vi "OAT State Machine Generate Event for Numeric.vi"(1 "Initialize":bool, 2 "Numeric":dbl format="%.2f", 4 "Enum":T1(ring) caption="Action") -> (7 "Event":bool)   [LabVIEW 2017]
doc: "Detects events for the numeric objects. The event of numeric range from changed, zero crossing,sign reversed and so on. When the event detected, the coresponding output is TRUE."
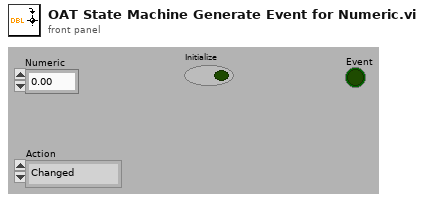
[diagram p1: front panel]
types:
  T1 = enum16{"Changed", ">0 to <0", "<0 to >0", ">0 to <=0", "<=0 to >0", ">=0 to <0", "<0 to >=0", ">0 to =0", "=0 to >0", "<0 to =0", "=0 to <0", "=0", "Zero Crossing", "Sign Reversed"}
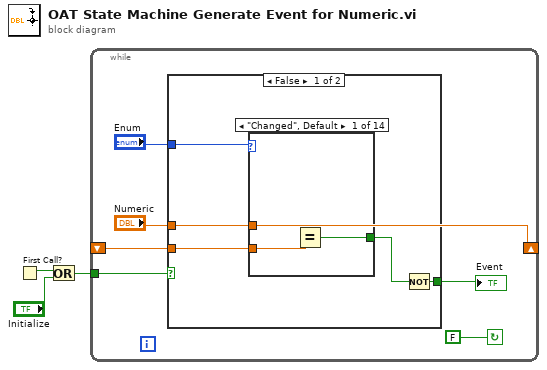
[diagram p0: block diagram]
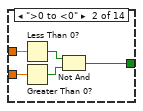
[diagram p2: hidden frame]
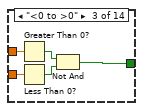
[diagram p3: hidden frame]
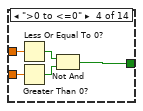
[diagram p4: hidden frame]
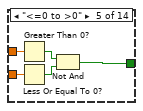
[diagram p5: hidden frame]
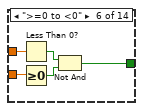
[diagram p6: hidden frame]
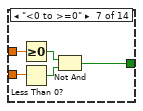
[diagram p7: hidden frame]
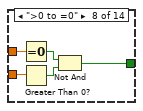
[diagram p8: hidden frame]
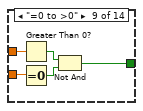
[diagram p9: hidden frame]
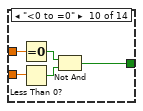
[diagram p10: hidden frame]
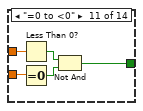
[diagram p11: hidden frame]
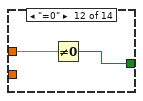
[diagram p12: hidden frame]
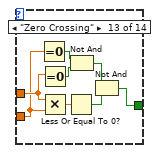
[diagram p13: hidden frame]
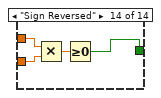
[diagram p14: hidden frame]
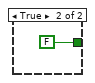
[diagram p15: hidden frame]
diagram:
  n1 = First Call?() -> (First Call?: T/F=w2:bool)
  n2 = Or(x=w2, y="Initialize") -> (x .or. y?=w3:bool)
  n3 = while {
    tunnel: w3 -> [w7]
    shift-left: _ -> [w9]
    shift-right: ["Numeric"] -> _
    stop <- FALSE continue-if-true
    n4 = case shown="False" w7 {
      tunnel: "Enum" -> [w14 _]
      tunnel: w9 -> [w13 _]
      tunnel: "Numeric" -> [w12 _]
      tunnel: [w10 FALSE] -> w5
      frame False {
        n5 = case shown="\"Changed\", Default" w14 {
          tunnel: w12 -> [w17 w22 w27 w32 w37 w41 w46 w51 w56 w61 w66 w69 w76 w80]
          tunnel: w13 -> [w16 w21 w26 w31 w36 w42 w47 w52 w57 w62 w67 _ w75 w81]
          tunnel: [w15 w18 w23 w28 w33 w38 w43 w48 w53 w58 w63 w68 w72 w78] -> w11
          frame "Changed", Default {
            n6 = Equal?(x=w17, y=w16) -> (x = y?=w15:bool)
          }
          frame ">0 to <0" {
            n7 = Less Than 0?(x=w22) -> (x < 0?=w19:bool)
            n8 = Greater Than 0?(x=w21) -> (x > 0?=w20:bool)
            n9 = Not And(1:w20, 2:w19) -> (0:w18:bool)
          }
          frame "<0 to >0" {
            n10 = Greater Than 0?(x=w27) -> (x > 0?=w25:bool)
            n11 = Less Than 0?(x=w26) -> (x < 0?=w24:bool)
            n12 = Not And(1:w24, 2:w25) -> (0:w23:bool)
          }
          frame ">0 to <=0" {
            n13 = Less Or Equal To 0?(x=w32) -> (x <= 0?=w30:bool)
            n14 = Greater Than 0?(x=w31) -> (x > 0?=w29:bool)
            n15 = Not And(1:w29, 2:w30) -> (0:w28:bool)
          }
          frame "<=0 to >0" {
            n16 = Greater Than 0?(x=w37) -> (x > 0?=w35:bool)
            n17 = Less Or Equal To 0?(x=w36) -> (x <= 0?=w34:bool)
            n18 = Not And(1:w34, 2:w35) -> (0:w33:bool)
          }
          frame ">=0 to <0" {
            n19 = Less Than 0?(x=w41) -> (x < 0?=w40:bool)
            n20 = Greater Or Equal To 0?(x=w42) -> (x >= 0?=w39:bool)
            n21 = Not And(1:w39, 2:w40) -> (0:w38:bool)
          }
          frame "<0 to >=0" {
            n22 = Greater Or Equal To 0?(x=w46) -> (x >= 0?=w45:bool)
            n23 = Less Than 0?(x=w47) -> (x < 0?=w44:bool)
            n24 = Not And(1:w44, 2:w45) -> (0:w43:bool)
          }
          frame ">0 to =0" {
            n25 = Equal To 0?(x=w51) -> (x = 0?=w50:bool)
            n26 = Greater Than 0?(x=w52) -> (x > 0?=w49:bool)
            n27 = Not And(1:w49, 2:w50) -> (0:w48:bool)
          }
          frame "=0 to >0" {
            n28 = Greater Than 0?(x=w56) -> (x > 0?=w55:bool)
            n29 = Equal To 0?(x=w57) -> (x = 0?=w54:bool)
            n30 = Not And(1:w54, 2:w55) -> (0:w53:bool)
          }
          frame "<0 to =0" {
            n31 = Equal To 0?(x=w61) -> (x = 0?=w60:bool)
            n32 = Less Than 0?(x=w62) -> (x < 0?=w59:bool)
            n33 = Not And(1:w59, 2:w60) -> (0:w58:bool)
          }
          frame "=0 to <0" {
            n34 = Less Than 0?(x=w66) -> (x < 0?=w65:bool)
            n35 = Equal To 0?(x=w67) -> (x = 0?=w64:bool)
            n36 = Not And(1:w64, 2:w65) -> (0:w63:bool)
          }
          frame "=0" {
            n37 = Not Equal To 0?(x=w69) -> (x != 0?=w68:bool)
          }
          frame "Zero Crossing" {
            n38 = Equal To 0?(x=w75) -> (x = 0?=w73:bool)
            n39 = Equal To 0?(x=w76) -> (x = 0?=w74:bool)
            n40 = Multiply(x=w76, y=w75) -> (x*y=w77:dbl)
            n41 = Less Or Equal To 0?(x=w77) -> (x <= 0?=w70:bool)
            n42 = Not And(1:w74, 2:w73) -> (0:w71:bool)
            n43 = Not And(1:w70, 2:w71) -> (0:w72:bool)
          }
          frame "Sign Reversed" {
            n44 = Multiply(x=w80, y=w81) -> (x*y=w79:dbl)
            n45 = Greater Or Equal To 0?(x=w79) -> (x >= 0?=w78:bool)
          }
        }
        n46 = Not(x=w11) -> (.not. x?=w10:bool)
      }
      frame True {
      }
    }
    "Event" <- w5
  }
